vi "Debug Logger Client.vi"(8 "error in (no error)":errorcluster, 10 "Message":string, 11 "Debug Type":T1) -> (0 "error out":errorcluster)   [LabVIEW 2013]
uses:
  Debug Type.ctl
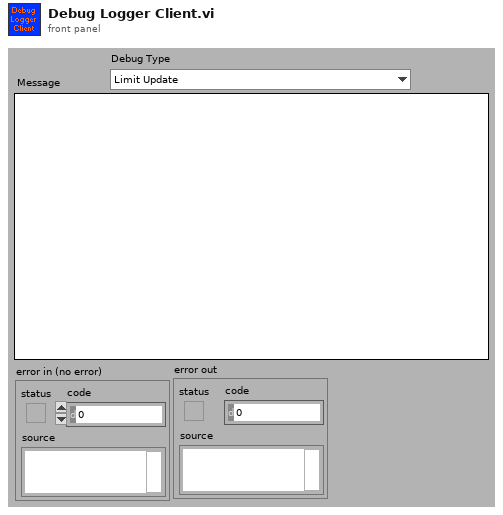
[diagram p1: front panel]
types:
  T1 = typedef "Debug Type.ctl" = enum16{"Limit Update", "Limit Change", ""}
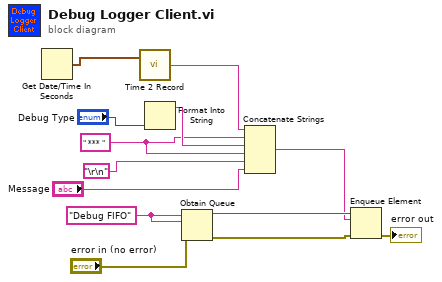
[diagram p0: block diagram]
diagram:
  w10 = " *** " ("string")
  w13 = "Debug FIFO" ("name (unnamed)")
  n1 = Get Date/Time In Seconds() -> (seconds since 1Jan1904=w7:timestamp)
  n2 = call "Time 2 Record.vi"("Time Stamp"=w7) -> ("String"=w6:string)  [unwired: 1 in]
  n3 = Format Into String("Debug Type") -> (resulting string=w11:string)  [unwired: 3 in, 1 out]
  n4 = Obtain Queue(name (unnamed)=w13, element data type=w13, error in (no error)="error in (no error)") -> (queue out=w4:refnum<queue>, error out=w5:errorcluster)  [unwired: 2 in, 1 out]
  n5 = Concatenate Strings(w6, w10, w11, w10, "\r\n", "Message") -> (w3:string)
  n6 = Enqueue Element(queue=w4, element=w3, error in (no error)=w5) -> (error out=→"error out":errorcluster)  [unwired: 1 in, 2 out]
